vi "Tune And Test Arm.vi"() -> ()   [LabVIEW 2018]
uses:
  <vilib>/Rock Robotics/WPI/ThirdParty/Phoenix-LabVIEW/Motor Controller/Controls/CTRE_Phoenix_MotorControl_FeedbackDevice.ctl
  <vilib>/Rock Robotics/WPI/ThirdParty/Phoenix-LabVIEW/Motor Controller/Controls/CTRE_Phoenix_MotorControl_LimitSwitchSource_Local.ctl
  <vilib>/Rock Robotics/WPI/ThirdParty/Phoenix-LabVIEW/Motor Controller/Controls/CTRE_Phoenix_MotorControl_LimitSwitchNormal.ctl
  <vilib>/Rock Robotics/WPI/ThirdParty/Phoenix-LabVIEW/Motor Controller/Controls/CTRE_Phoenix_MotorControl_StatusFrameEnhanced.ctl
  <vilib>/Rock Robotics/WPI/ThirdParty/Phoenix-LabVIEW/Motor Controller/Controls/CTRE_Phoenix_MotorControl_VelocityMeasurementPeriod.ctl
  <vilib>/Rock Robotics/WPI/ThirdParty/Phoenix-LabVIEW/Motor Controller/Controls/CTRE_Phoenix_MotorControl_ControlMode.ctl
  <extravilib>/ChannelInstances/Lossy Stream-c(i32,i32,i32,i32)/Read With Abort.vi
  <extravilib>/ChannelInstances/Lossy Stream-c(i32,i32,i32,i32)/Write With Abort.vi
  <extravilib>/ChannelInstances/Lossy Stream-c(i32,i32,i32,i32)/EndpointRead.vi
  <extravilib>/ChannelInstances/Lossy Stream-c(i32,i32,i32,i32)/Endpoint.vi
  <extravilib>/ChannelInstances/Lossy Stream-c(i32,i32,i32,i32)/Instantiate.vi
  <extravilib>/ChannelInstances/Lossy Stream-c(i32,i32,i32,i32)/)Channel.vi
  <resource>/ChannelSupport/_ChannelSupport/WaitIfNeeded.vi
  <vilib>/Rock Robotics/WPI/ThirdParty/Phoenix-LabVIEW/Motor Controller/Get/CTRE_Phoenix_MotorController_GetSelectedSensorData.vi
  <extravilib>/ChannelInstances/Lossy Stream-c(i32,i32,i32,i32).lvlib
panel:
  in  "A? or B":bool=TRUE
  in  "Height B":dbl=70.0
  in  "Zero Sensor":bool
  in  "Height A":dbl=10.0
  in  "Do Motion Magic":bool=TRUE
  in  "Go Down Direction":bool
  out "Velocity":cluster{"Output":dbl, "Velocity":i32}(graph)
  out "Position":cluster{"Target Position":i32, "Position":i32}(graph)={"Target Position"=0, "Position"=1}
  in  "Gravity Compensator":dbl=0.038
  in  "Output":dbl=0.1
  in  "F":dbl=11.9
  in  "D":dbl
  in  "I":dbl
  in  "P":dbl
  in  "Acceleration":i32=60
  in  "Cruise Velocity":i32=40
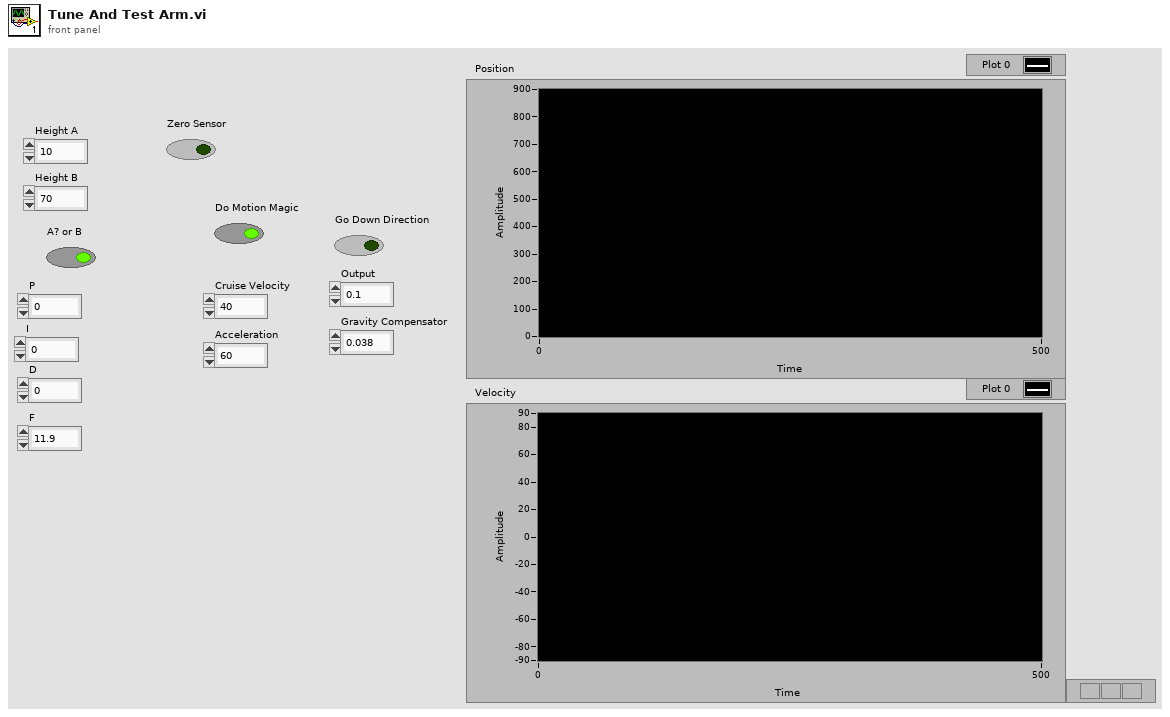
[diagram p1: front panel]
types:
  T1 = typedef "CTRE_Phoenix_MotorControl_StatusFrameEnhanced.ctl" = u16
  T2 = typedef "CTRE_Phoenix_MotorControl_VelocityMeasurementPeriod.ctl" = u16
  T3 = typedef "CTRE_Phoenix_MotorControl_LimitSwitchNormal.ctl" = enum16{"Normally Open", "Normally Closed", "Disabled"}
  T4 = typedef "CTRE_Phoenix_MotorControl_LimitSwitchSource_Local.ctl" = enum16{"Feedback Connector", "Remote Talon SRX", "Remote CANifier", "Deactivated"}
  T5 = typedef "CTRE_Phoenix_MotorControl_FeedbackDevice.ctl" = i8
  T6 = typedef "WPI_MotorControlDeviceRef.ctl" = cluster{"DeviceStatus":errorcluster, "Type":T7, "PWM":cluster{"PWM Channel":T8, "DeadBand":T9}, "CAN":cluster{"Device Number":u8, "SetOutput VI Ref":variant, "GetOutput VI Ref":variant, "Enable VI Ref":variant, "Disable VI Ref":variant, "Data":variant}, "Invert":bool, "DIO PWM":cluster{"PWM \"Enable\" Channel":T8, "DIOChannel":T10, "PWM Rate":dbl}}
  T7 = typedef "WPI_MotorControlType.ctl" = enum16{"PWM", "CAN", "DIO PWM"}
  T8 = typedef "FPGA_DIOPWMChannel.ctl" = enum8{"PWM 0", "PWM 1", "PWM 2", "PWM 3", "PWM 4", "PWM 5", "PWM 6", "PWM 7", "PWM 8", "PWM 9", "PWM MXP 0", "PWM MXP 1", "PWM MXP 2", "PWM MXP 3", "PWM MXP 4", "PWM MXP 5", "PWM MXP 6", "PWM MXP 7", "PWM MXP 8", "PWM MXP 9", "Invalid"}
  T9 = typedef "WPI_PWMDeadband.ctl" = cluster{"Name":string, "maxPositivePwm":i32, "minPositivePwm":i32, "centerPwm":i32, "maxNegativePwm":i32, "minNegativePwm":i32, "angularRange":u16}
  T10 = typedef "FPGA_DIOChannel.ctl" = enum8{"DIO 0", "DIO 1", "DIO 2", "DIO 3", "DIO 4", "DIO 5", "DIO 6", "DIO 7", "DIO 8", "DIO 9", "DIO MXP 0", "DIO MXP 1", "DIO MXP 2", "DIO MXP 3", "DIO MXP 4", "DIO MXP 5", "DIO MXP 6", "DIO MXP 7", "DIO MXP 8", "DIO MXP 9", "DIO MXP 10", "DIO MXP 11", "DIO MXP 12", "DIO MXP 13", "DIO MXP 14", "DIO MXP 15", "SPI Port CS1", "SPI Port CS2", "SPI Port CS3", "SPI Port MISO", "SPI Port MOSI", "Invalid"}
  T11 = cluster{"Position":i32, "Velocity":i32, "Target Position":i32, "Target Velocity":i32}
  T12 = typedef "Lossy Stream-c(i32,i32,i32,i32).lvlib/)Channel.ctl" = refnum<queue>
  T13 = enum16{"DemandType_Neutral", "DemandType_AuxPID", "DemandType_ArbitraryFeedForward"}
  T14 = typedef "CTRE_Phoenix_MotorControl_ControlMode.ctl" = u16
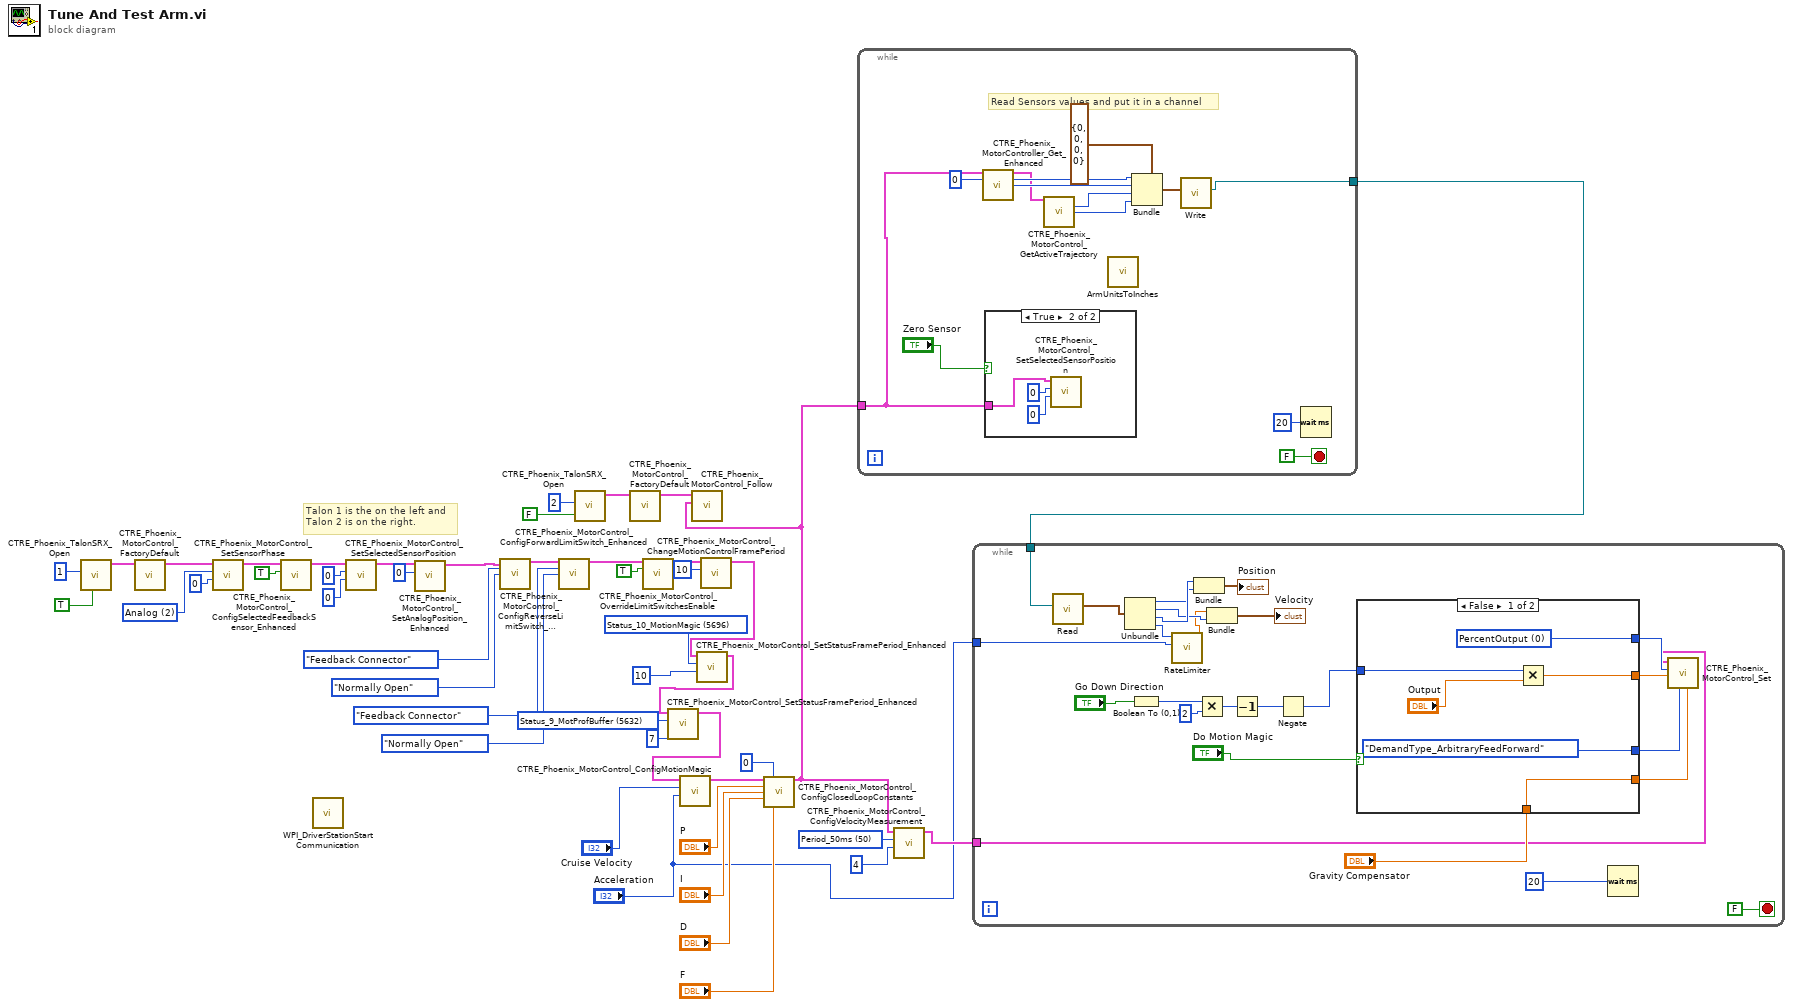
[diagram p0: block diagram]
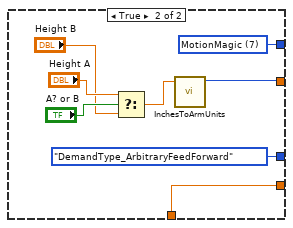
[diagram p2: hidden frame]
diagram:
  w6 = T1 5632 items=["Status_1_General"=5120, "Status_2_Feedback0"=5184, "Status_3_Quadrature"=5248, "Status_4_AinTempVbat"=5312, "Status_6_Misc"=5440, "Status_7_CommStatus"=5504, "Status_8_PulseWidth"=5568, "Status_9_MotProfBuffer"=5632, "Status_10_MotionMagic"=5696, "Status_11_UartGadgeteer"=5760, "Status_12_Feedback1"=5824, "Status_13_Base_PIDF0"=5888, "Status_14_Turn_PIDF1"=5952, "Status_15_FirmwareApiStatus"=6016] ("Status Frame")
  w13 = T2 50 items=["Period_1ms"=1, "Period_2ms"=2, "Period_5ms"=5, "Period_10ms"=10, "Period_20ms"=20, "Period_25ms"=25, "Period_50ms"=50, "Period_100ms"=100] ("Velocity Measurement Period")
  w16 = T1 5696 items=["Status_1_General"=5120, "Status_2_Feedback0"=5184, "Status_3_Quadrature"=5248, "Status_4_AinTempVbat"=5312, "Status_6_Misc"=5440, "Status_7_CommStatus"=5504, "Status_8_PulseWidth"=5568, "Status_9_MotProfBuffer"=5632, "Status_10_MotionMagic"=5696, "Status_11_UartGadgeteer"=5760, "Status_12_Feedback1"=5824, "Status_13_Base_PIDF0"=5888, "Status_14_Turn_PIDF1"=5952, "Status_15_FirmwareApiStatus"=6016] ("Status Frame")
  w42 = T5 2 items=["QuadEncoder"=0, "Analog"=2, "Tachometer"=4, "Pulse Width Encoded Position"=8, "Sensor Sum (S0 + S1)"=9, "Sensor Difference (D0 - D1)"=10, "Remote Source 0"=11, "Remote Source 1"=12, "Software Emulated"=15] ("Feedback Device")
  # "Talon 1 is the on the left and\nTalon 2 is on the right."
  n1 = call <vilib>:"CTRE_Phoenix_TalonSRX_Open.vi"("Invert"=TRUE, "Device Number"=u8 1) -> ("CAN Talon SRX Ref"=w46:T6)  [unwired: 8 in, 1 out]
  n2 = call <vilib>:"CTRE_Phoenix_MotorControl_FactoryDefault.vi"("PhoenixMotorControlDevRef"=w46) -> ("PhoenixMotorControlDevRef"=w43:T6)  [unwired: 9 in, 1 out]
  n3 = call <vilib>:"CTRE_Phoenix_MotorControl_ConfigSelectedFeedbackSensor_Enhanced.vi"("pidLoopIdx"=0, "Feedback Device"=w42, "PhoenixMotorControlDevRef"=w43) -> ("PhoenixMotorControlDevRef"=w29:T6)  [unwired: 7 in, 1 out]
  n4 = call <vilib>:"CTRE_Phoenix_MotorControl_SetSensorPhase.vi"("PhaseSensor"=TRUE, "PhoenixMotorControlDevRef"=w29) -> ("PhoenixMotorControlDevRef"=w27:T6)  [unwired: 8 in, 1 out]
  n5 = call <vilib>:"WPI_DriverStationStart Communication.vi"() -> ()  [unwired: 12 in]
  n6 = call <vilib>:"CTRE_Phoenix_MotorControl_SetSelectedSensorPosition.vi"("pidLoopIdx"=u32 0, "New Sensor Position"=0, "PhoenixMotorControlDevRef"=w27) -> ("PhoenixMotorControlDevRef"=w3:T6)  [unwired: 7 in, 1 out]
  n7 = call <vilib>:"CTRE_Phoenix_MotorControl_SetAnalogPosition_Enhanced.vi"("New Position"=0, "PhoenixMotorControlDevRef"=w3) -> ("PhoenixMotorControlDevRef"=w2:T6)  [unwired: 8 in, 1 out]
  n8 = call <vilib>:"CTRE_Phoenix_MotorControl_ConfigReverseLimitSwitch_Enhanced.vi"("PhoenixMotorControlDevRef"=w2, "Limit Switch Source"=CTRE_Phoenix_MotorControl_LimitSwitchSource_Local."Feedback Connector", "NormallyOpenOrClosed"=CTRE_Phoenix_MotorControl_LimitSwitchNormal."Normally Open") -> ("PhoenixMotorControlDevRef"=w38:T6)  [unwired: 11 in, 1 out]
  n9 = call <vilib>:"CTRE_Phoenix_MotorControl_ConfigForwardLimitSwitch_Enhanced.vi"("PhoenixMotorControlDevRef"=w38, "Limit Switch Source"=CTRE_Phoenix_MotorControl_LimitSwitchSource_Local."Feedback Connector", "NormallyOpenOrClosed"=CTRE_Phoenix_MotorControl_LimitSwitchNormal."Normally Open") -> ("PhoenixMotorControlDevRef"=w33:T6)  [unwired: 11 in, 1 out]
  n10 = call <vilib>:"CTRE_Phoenix_TalonSRX_Open.vi"("Invert"=FALSE, "Device Number"=u8 2) -> ("CAN Talon SRX Ref"=w44:T6)  [unwired: 8 in, 1 out]
  n11 = call <vilib>:"CTRE_Phoenix_MotorControl_FactoryDefault.vi"("PhoenixMotorControlDevRef"=w44) -> ("PhoenixMotorControlDevRef"=w31:T6)  [unwired: 9 in, 1 out]
  n12 = call <vilib>:"CTRE_Phoenix_MotorControl_OverrideLimitSwitchesEnable.vi"("PhoenixMotorControlDevRef"=w33, "Override Limit Switch Enable?"=TRUE) -> ("PhoenixMotorControlDevRef"=w11:T6)  [unwired: 12 in, 1 out]
  n13 = call <vilib>:"CTRE_Phoenix_MotorControl_ChangeMotionControlFramePeriod.vi"("periodMs"=10, "PhoenixMotorControlDevRef"=w11) -> ("PhoenixMotorControlDevRef"=w10:T6)  [unwired: 8 in, 1 out]
  n14 = call <vilib>:"CTRE_Phoenix_MotorControl_SetStatusFramePeriod_Enhanced.vi"("periodMs"=10, "Status Frame"=w16, "PhoenixMotorControlDevRef"=w10) -> ("PhoenixMotorControlDevRef"=w8:T6)  [unwired: 7 in, 1 out]
  n15 = call <vilib>:"CTRE_Phoenix_MotorControl_SetStatusFramePeriod_Enhanced.vi"("periodMs"=7, "Status Frame"=w6, "PhoenixMotorControlDevRef"=w8) -> ("PhoenixMotorControlDevRef"=w7:T6)  [unwired: 7 in, 1 out]
  n16 = call <vilib>:"CTRE_Phoenix_MotorControl_ConfigMotionMagic.vi"("Acceleration"="Acceleration", "Cruise Velocity"="Cruise Velocity", "PhoenixMotorControlDevRef"=w7) -> ("PhoenixMotorControlDevRef"=w23:T6)  [unwired: 7 in, 1 out]
  n17 = call <vilib>:"CTRE_Phoenix_MotorControl_ConfigClosedLoopConstants.vi"("PhoenixMotorControlDevRef"=w23, "slotIdx"=0, "P"="P", "I"="I", "D"="D", "F"="F") -> ("PhoenixMotorControlDevRef"=w18:T6)  [unwired: 8 in, 1 out]
  n18 = call <vilib>:"CTRE_Phoenix_MotorControl_Follow.vi"("Master Controller to Follow"=w18, "PhoenixMotorControlDevRef"=w31) -> ()  [unwired: 8 in, 2 out]
  n19 = while {
    tunnel: [w51] -> w30
    tunnel: w18 -> [w50]
    stop <- FALSE stop-if-true
    # "Read Sensors values and put it in a channel"
    n20 = call-poly <vilib>:"CTRE_Phoenix_MotorController_Get_Enhanced.vi"("PhoenixMotorControlDevRef"=w50, "pidLoopIdx"=u32 0) -> ("PhoenixMotorControlDevRef"=w49:T6, "Position (Raw Sensor Units)"=w57:i32, "Velocity (Raw Sensor Units per 100 ms)"=w56:i32)  [unwired: 10 in, 1 out]
    n21 = case shown="True" "Zero Sensor" {
      tunnel: w50 -> [_ w61]
      frame False {
      }
      frame True {
        n22 = call <vilib>:"CTRE_Phoenix_MotorControl_SetSelectedSensorPosition.vi"("pidLoopIdx"=u32 0, "New Sensor Position"=0, "PhoenixMotorControlDevRef"=w61) -> ()  [unwired: 7 in, 2 out]
      }
    }
    n23 = call <vilib>:"CTRE_Phoenix_MotorControl_GetActiveTrajectory.vi"("PhoenixMotorControlDevRef"=w49) -> ("Position (Sensor Units)"=w53:i32, "Velocity (Sensor Units per 100 ms)"=w48:i32)  [unwired: 10 in, 3 out]
    n24 = call "ArmUnitsToInches.vi"() -> ()  [unwired: 10 in, 2 out]
    n25 = Bundle(cluster=T11 {"Position"=0, "Velocity"=0, "Target Position"=0, "Target Velocity"=0} ("Sensor Data"), "Position"=w57, "Velocity"=w56, "Target Position"=w53, "Target Velocity"=w48) -> (w52:T11)
    n26 = call <extravilib>:"Write.vi"("element"=w52) -> ("channel"=w51:T12)  [unwired: 8 in, 2 out]
    n27 = Wait (ms)(milliseconds to wait=u32 20) -> ()  [unwired: 1 out]
  }
  n28 = call <vilib>:"CTRE_Phoenix_MotorControl_ConfigVelocityMeasurement.vi"("Window Size"=4, "Velocity Measurement Period"=w13, "PhoenixMotorControlDevRef"=w18) -> ("PhoenixMotorControlDevRef"=w12:T6)  [unwired: 7 in, 1 out]
  n29 = while {
    tunnel: w30 -> [w74]
    tunnel: w12 -> [w67]
    tunnel: "Acceleration" -> [w64]
    stop <- FALSE stop-if-true
    n30 = call <extravilib>:"Read.vi"("channel"=w74) -> ("element"=w73:T11)  [unwired: 5 in, 5 out]
    n31 = Unbundle(w73) -> ("Position"=w71:i32, "Velocity"=w69:i32, "Target Position"=w72:i32, "Target Velocity"=w66:i32)
    n32 = Boolean To (0,1)(Boolean="Go Down Direction") -> (0, 1=w85:i16)
    n33 = call "RateLimiter.vi"("Max dx/dt"=w64, "Input"=w66) -> ("Output"=w65:dbl)  [unwired: 9 in]
    n34 = Bundle("Target Position"=w72, "Position"=w71) -> (→"Position":cluster{"Target Position":i32, "Position":i32})  [unwired: 1 in]
    n35 = Multiply(x=w85, y=i16 2) -> (x*y=w83:i16)
    n36 = Bundle("Output"=w65, "Velocity"=w69) -> (→"Velocity":cluster{"Output":dbl, "Velocity":i32})  [unwired: 1 in]
    n37 = Decrement(x=w83) -> (x-1=w82:i16)
    n38 = Negate(x=w82) -> (-x=w81:i16)
    n39 = case shown="False" "Do Motion Magic" {
      tunnel: w81 -> [w94 _]
      tunnel: [T13."DemandType_ArbitraryFeedForward" ("DemandType") T13."DemandType_ArbitraryFeedForward" ("DemandType")] -> w79
      tunnel: [w92 w99] -> w78
      tunnel: [w91 w102] -> w77
      tunnel: [w90 w100] -> w76
      tunnel: "Gravity Compensator" -> [w90 w100]
      frame False {
        w91 = T14 0 items=["PercentOutput"=0, "Position"=1, "Velocity"=2, "Current"=3, "Follower"=5, "MotionProfile"=6, "MotionMagic"=7, "MotionProfileArc"=10, "Disabled"=15] ("Control Mode")
        n40 = Multiply(x=w94, y="Output") -> (x*y=w92:dbl)
      }
      frame True {
        w102 = T14 7 items=["PercentOutput"=0, "Position"=1, "Velocity"=2, "Current"=3, "Follower"=5, "MotionProfile"=6, "MotionMagic"=7, "MotionProfileArc"=10, "Disabled"=15] ("Control Mode")
        n41 = Select(t="Height A", s="A? or B", f="Height B") -> (s? t:f=w95:dbl)
        n42 = call "InchesToArmUnits.vi"("Inches"=w95) -> ("Sensor Units"=w99:i32)  [unwired: 10 in]
      }
    }
    n43 = Wait (ms)(milliseconds to wait=u32 20) -> ()  [unwired: 1 out]
    n44 = call <vilib>:"CTRE_Phoenix_MotorControl_Set.vi"("Demand1"=w76, "DemandType"=w79, "Output"=w78, "Control Mode"=w77, "PhoenixMotorControlDevRef"=w67) -> ()  [unwired: 5 in, 2 out]
  }
